vi "Parse Response Message.vi"(8 "error in":errorcluster, 11 "Axis in":refnum<class "Axis.lvclass">) -> (0 "error out":errorcluster, 3 "Axis out":refnum<class "Axis.lvclass">)   [LabVIEW 2018, in "Axis.lvlib" / "Axis.lvclass"]
doc: "This VI is in charge of querying and updating all the information about the Axis. This includes Position, Home Status, Moving Status, and whether there have been errors."
uses:
  Axis.lvclass
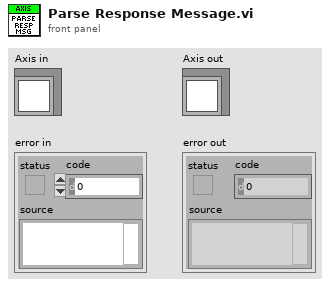
[diagram p1: front panel]
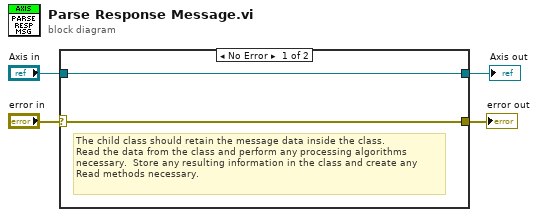
[diagram p0: block diagram]
diagram:
  n1 = case shown="No Error" "error in" {
    selector: "error in" -> [w5 w8]
    tunnel: [w5 w8] -> w3
    tunnel: [w6 w7] -> w1
    tunnel: "Axis in" -> [w6 w7]
    frame No Error {
      # "The child class should retain the message data inside the class.  \nRead the data from the class and perform any processing algorithms \nnecessary.  Store any resulting information in the class and create any \nRead methods necessary."
    }
    frame Error {
    }
  }
  "error out" <- w3
  "Axis out" <- w1
